vi "Compass on GIC 4.vi"(1 "GIC Input":T1={"Real/Sim"=FALSE, "WP Lats and Longs"={"WP Lats"=[], "WP Longs"=[]}, "GPS Time Int"=0.0, "GPS Com Port"="", "Compass Com Port"="", "Prop Com Port"="", "GPS Data"=[], "Compass"=0.0, "LMS Vector"=[], "Vision Vector"=[], "Direction Cmd"=0.0, "Speed Cmd"=0.0, "Time of Last GPS"=0.0, "WP Vector"=[], "WP Number"=0, "Num of WPs"=0, "SW Map"=[], "Obst Lats and Longs"={"Obst Lats"=[], "Obst Longs"=[]}, "Parameters"=[], "Path Cluster"={"Path x nodes"=[], "Path y nodes"=[]}, "     Use ?\nOff       On"=[TRUE, TRUE, FALSE, FALSE]} {"Obst Lats and Longs"."Obst Longs" format="%#_8g"; "Obst Lats and Longs"."Obst Lats" format="%#_8g"}) -> (0 "GIC Output":T1={"Real/Sim"=FALSE, "WP Lats and Longs"={"WP Lats"=[], "WP Longs"=[]}, "GPS Time Int"=0.0, "GPS Com Port"="", "Compass Com Port"="", "Prop Com Port"="", "GPS Data"=[], "Compass"=0.0, "LMS Vector"=[], "Vision Vector"=[], "Direction Cmd"=0.0, "Speed Cmd"=0.0, "Time of Last GPS"=0.0, "WP Vector"=[], "WP Number"=0, "Num of WPs"=0, "SW Map"=[], "Obst Lats and Longs"={"Obst Lats"=[], "Obst Longs"=[]}, "Parameters"=[], "Path Cluster"={"Path x nodes"=[], "Path y nodes"=[]}, "     Use ?\nOff       On"=[TRUE, TRUE, FALSE, FALSE]} {"Obst Lats and Longs"."Obst Longs" format="%#_8g"; "Obst Lats and Longs"."Obst Lats" format="%#_8g"})   [LabVIEW 2014]
panel:
  out "compass out":dbl
  # "GPS"
  # "LMS"
  # "Vision"
  # "Prop"
  # "GPS"
  # "LMS"
  # "Vision"
  # "Prop"
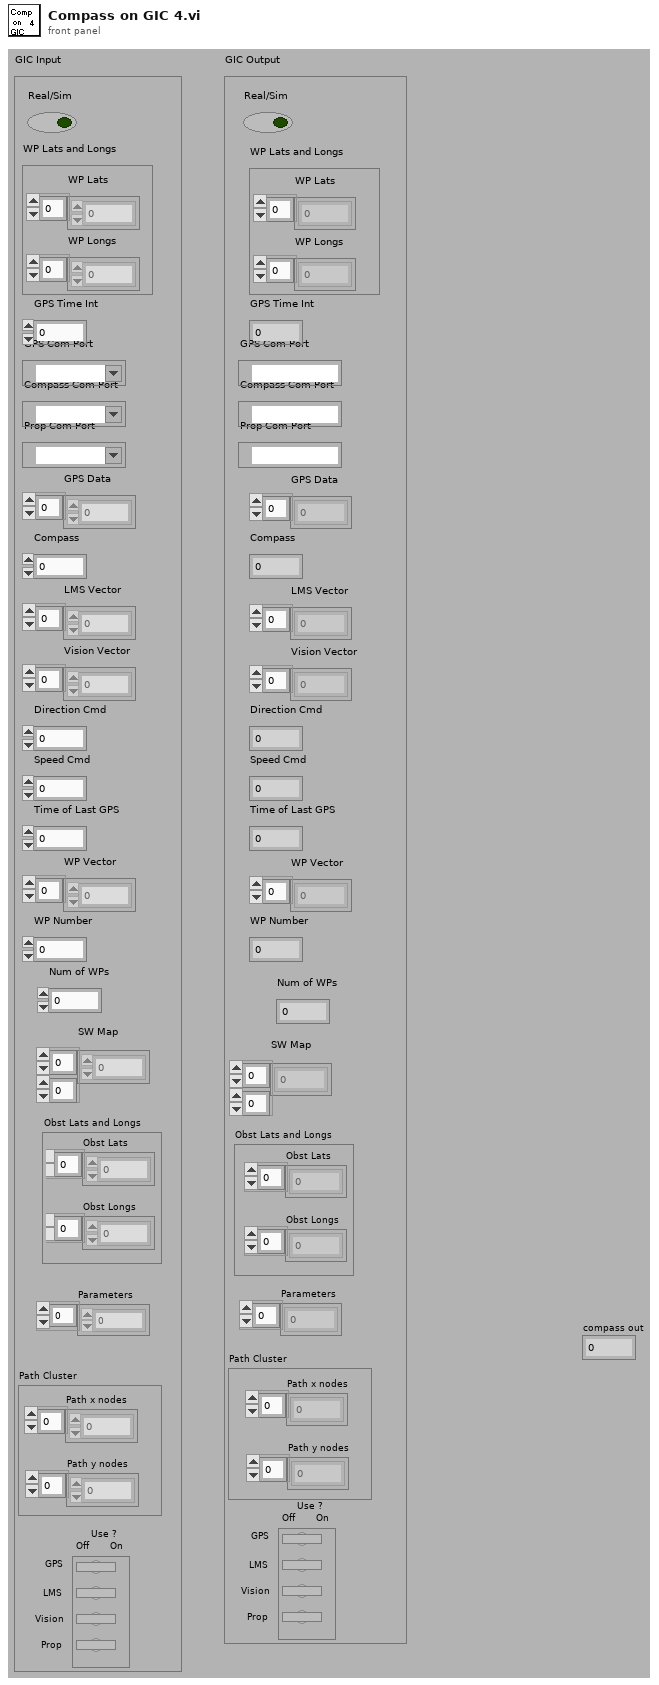
[diagram p1: front panel]
types:
  T1 = cluster{"Real/Sim":bool, "WP Lats and Longs":cluster{"WP Lats":dbl[], "WP Longs":dbl[]}, "GPS Time Int":dbl, "GPS Com Port":refnum<visa-resource-name>, "Compass Com Port":refnum<visa-resource-name>, "Prop Com Port":refnum<visa-resource-name>, "GPS Data":dbl[], "Compass":dbl, "LMS Vector":dbl[], "Vision Vector":dbl[], "Direction Cmd":dbl, "Speed Cmd":dbl, "Time of Last GPS":dbl, "WP Vector":dbl[], "WP Number":i32, "Num of WPs":i16, "SW Map":i32[][], "Obst Lats and Longs":cluster{"Obst Lats":dbl[], "Obst Longs":dbl[]}, "Parameters":dbl[], "Path Cluster":cluster{"Path x nodes":dbl[], "Path y nodes":dbl[]}, "     Use ?\nOff       On":bool[]}
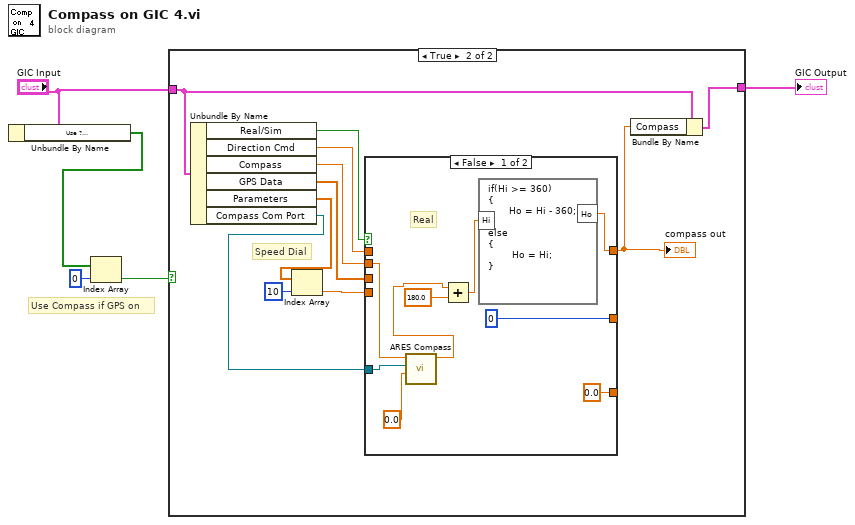
[diagram p0: block diagram]
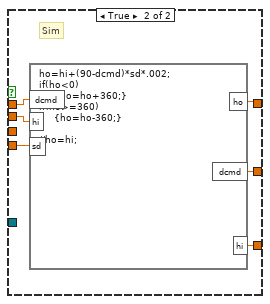
[diagram p3: hidden frame]
diagram:
  # "Use Compass if GPS on"
  n1 = Unbundle By Name("GIC Input") -> ("Use ?\nOff       On"=w3:bool[])
  n2 = Index Array(array=w3, index=0) -> (element=w1:bool)
  n3 = case shown="True" w1 {
    tunnel: "GIC Input" -> [w6 w12]
    tunnel: [w6 w11] -> w5
    frame False {
    }
    frame True {
      # "Speed Dial"
      n4 = Unbundle By Name(w12) -> ("Real/Sim"=w16:bool, "Direction Cmd"=w10:dbl, "Compass"=w9:dbl, "GPS Data"=w17:dbl[], "Parameters"=w15:dbl[], "Compass Com Port"=w7:refnum<visa-resource-name>)
      n5 = Index Array(array=w15, index=10) -> (element=w13:dbl)
      n6 = case shown="False" w16 {
        tunnel: w10 -> [_ w31]
        tunnel: w9 -> [w24 w30]
        tunnel: [w19 w32] -> w8
        tunnel: w17 -> [_ _]
        tunnel: w13 -> [_ w29]
        tunnel: [0 w28] -> _
        tunnel: [0.0 ("hi") w27] -> _
        tunnel: w7 -> [w23 _]
        frame False {
          # "Real"
          n7 = call "ARES Compass.vi"("Input time of last compass read"=0.0, "Compass Com Port"=w23, "Compass In"=w24) -> ("Compass Out"=w20:dbl)  [unwired: 6 in, 1 out]
          n8 = Add(x=w20, y=180.0) -> (x+y=w18:dbl)
          n9 = formula code="if(Hi >= 360)\n{\n       Ho = Hi - 360;\n}\nelse\n{\n        Ho = Hi;\n}"("Hi"=w18) -> ("Ho"=w19:dbl)
        }
        frame True {
          # "Sim"
          n10 = formula code="ho=hi+(90-dcmd)*sd*.002;\nif(ho<0)\n     {ho=ho+360;}\nif(ho>=360)\n     {ho=ho-360;}\n\n//ho=hi;"("dcmd"=w31, "hi"=w30, "sd"=w29) -> ("ho"=w32:dbl, "dcmd"=w28:dbl, "hi"=w27:dbl)
        }
      }
      "compass out" <- w8
      n11 = Bundle By Name(cluster=w12, "Compass"=w8) -> (w11:T1)
    }
  }
  "GIC Output" <- w5
